vi "TrajectoryTrend.vi"() -> ()   [LabVIEW 2023]
uses:
  <vilib>/Rock Robotics/Network Tables/NT Read Number.vi
  <vilib>/Rock Robotics/Network Tables/NT Read Boolean.vi
  Dash_Globals.vi
panel:
  out "Traj Chart":T1(graph)
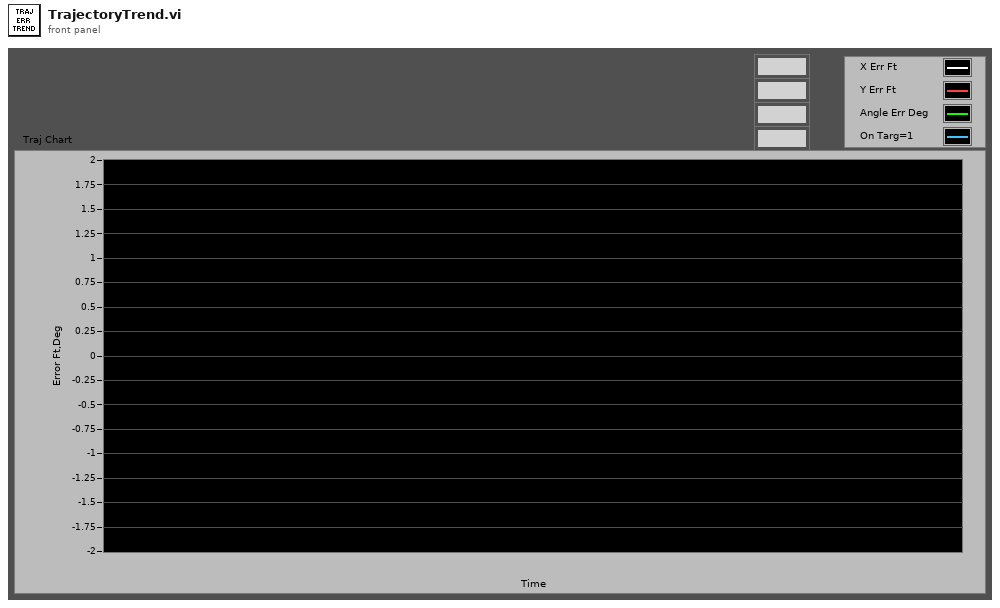
[diagram p1: front panel]
types:
  T1 = cluster{"value":dbl, "value":dbl, "value":dbl, dbl}
  T2 = enum8{"Tele-Op Disabled", "Tele-Op Enabled", "Auto Disabled", "Auto Enabled", "Test Disabled", "Test Enabled", "Disconnected", "No Code", "E-Stop"}
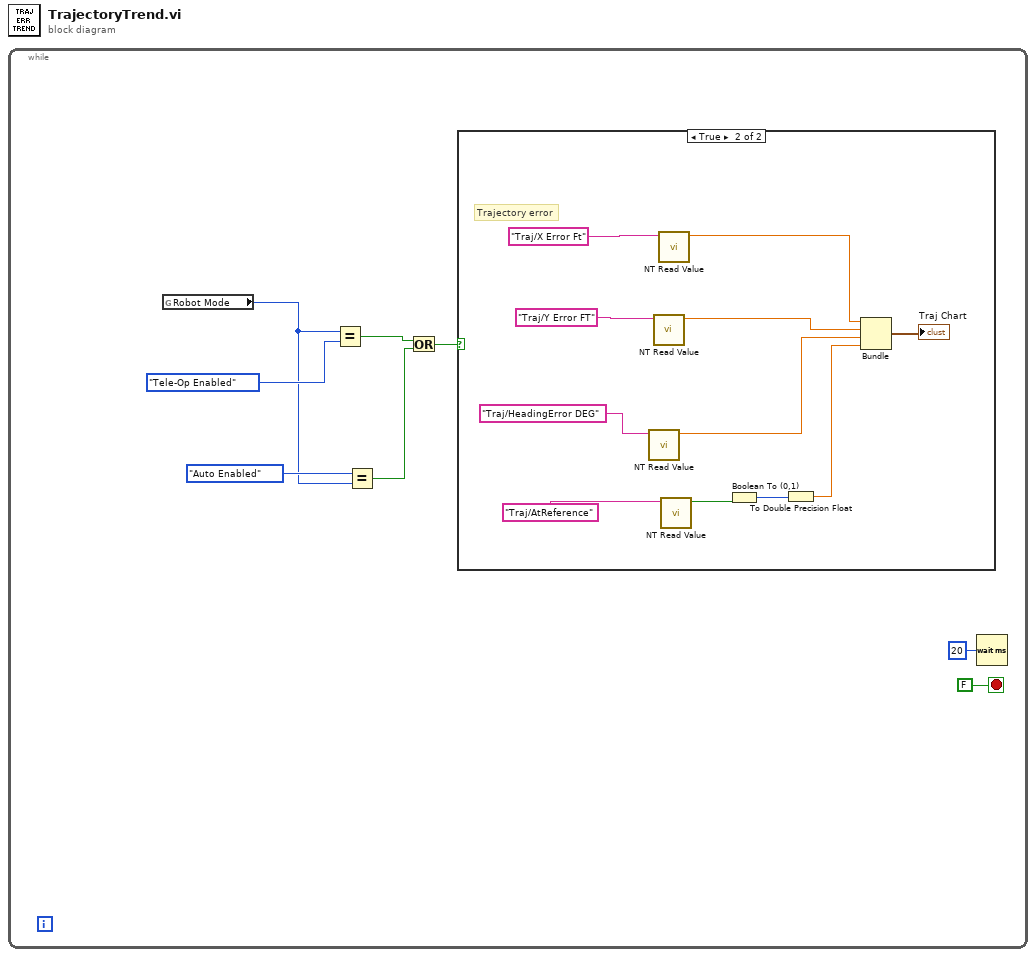
[diagram p0: block diagram]
diagram:
  n1 = while {
    stop <- FALSE stop-if-true
    n2 = global read "Dash_Globals.vi" "Robot Mode"() -> (w4:T2)
    n3 = Equal?(x=w4, y=T2."Tele-Op Enabled") -> (x = y?=w3:bool)
    n4 = Equal?(x=T2."Auto Enabled" ("y"), y=w4) -> (x = y?=w2:bool)
    n5 = Or(x=w3, y=w2) -> (x .or. y?=w1:bool)
    n6 = case shown="True" w1 {
      frame False {
      }
      frame True {
        # "Trajectory error"
        n7 = call-poly <vilib>:"NT Read Value.vi"("name"="Traj/HeadingError DEG" ("Name")) -> ("value"=w11:dbl)  [unwired: 8 in, 2 out]
        n8 = call-poly <vilib>:"NT Read Value.vi"("name"="Traj/Y Error FT" ("Name")) -> ("value"=w12:dbl)  [unwired: 8 in, 2 out]
        n9 = call-poly <vilib>:"NT Read Value.vi"("name"="Traj/X Error Ft" ("Name")) -> ("value"=w13:dbl)  [unwired: 8 in, 2 out]
        n10 = call-poly <vilib>:"NT Read Value.vi"("name"="Traj/AtReference" ("Name")) -> ("value"=w15:bool)  [unwired: 8 in, 2 out]
        n11 = Boolean To (0,1)(Boolean=w15) -> (0, 1=w14:i16)
        n12 = To Double Precision Float(number=w14) -> (double precision float=w10:dbl)
        n13 = Bundle("value"=w13, "value"=w12, "value"=w11, w10) -> (→"Traj Chart":T1)  [unwired: 1 in]
      }
    }
    n14 = Wait (ms)(milliseconds to wait=u32 20) -> ()  [unwired: 1 out]
  }
